vi "Scripting_AddVIInsideNoErrorCase.vi"(0 "ViToModify":refnum<vi>, 1 "VIToAdd":path=path "C:/GDS_Test/82/AO/NativeBase_class/protected/StartNP1.vi", 5 "error in (no error)":errorcluster, 6 "AddVIOnLeftSideCaseStructure":bool, 7 "OnlyReference":bool) -> (19 "error out":errorcluster)   [LabVIEW 2020]
uses:
  <vilib>/Utility/miscctls.llb/LVPointTypeDef.ctl
  <vilib>/Utility/miscctls.llb/LVPositionTypeDef.ctl
  <vilib>/Utility/miscctls.llb/LVRectTypeDef.ctl
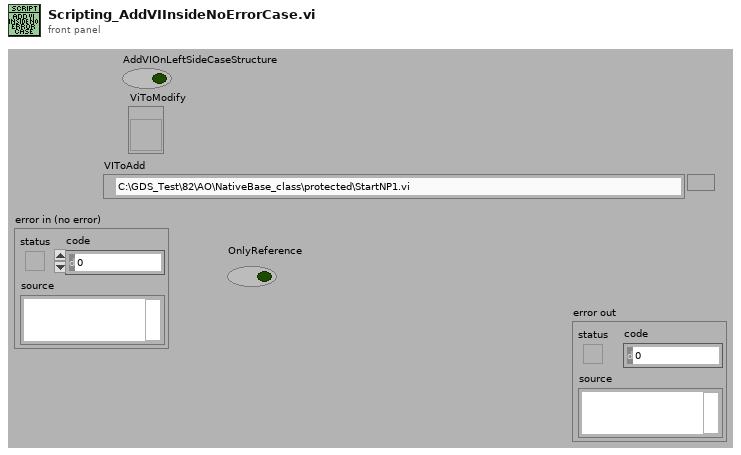
[diagram p1: front panel]
types:
  T1 = typedef "LVPositionTypeDef.ctl" = cluster{"Left":i32, "Top":i32}
  T2 = typedef "LVPointTypeDef.ctl" = cluster{"Horizontal":i16, "Vertical":i16}
  T3 = typedef "LVRectTypeDef.ctl" = cluster{"Left":i16, "Top":i16, "Right":i16, "Bottom":i16}
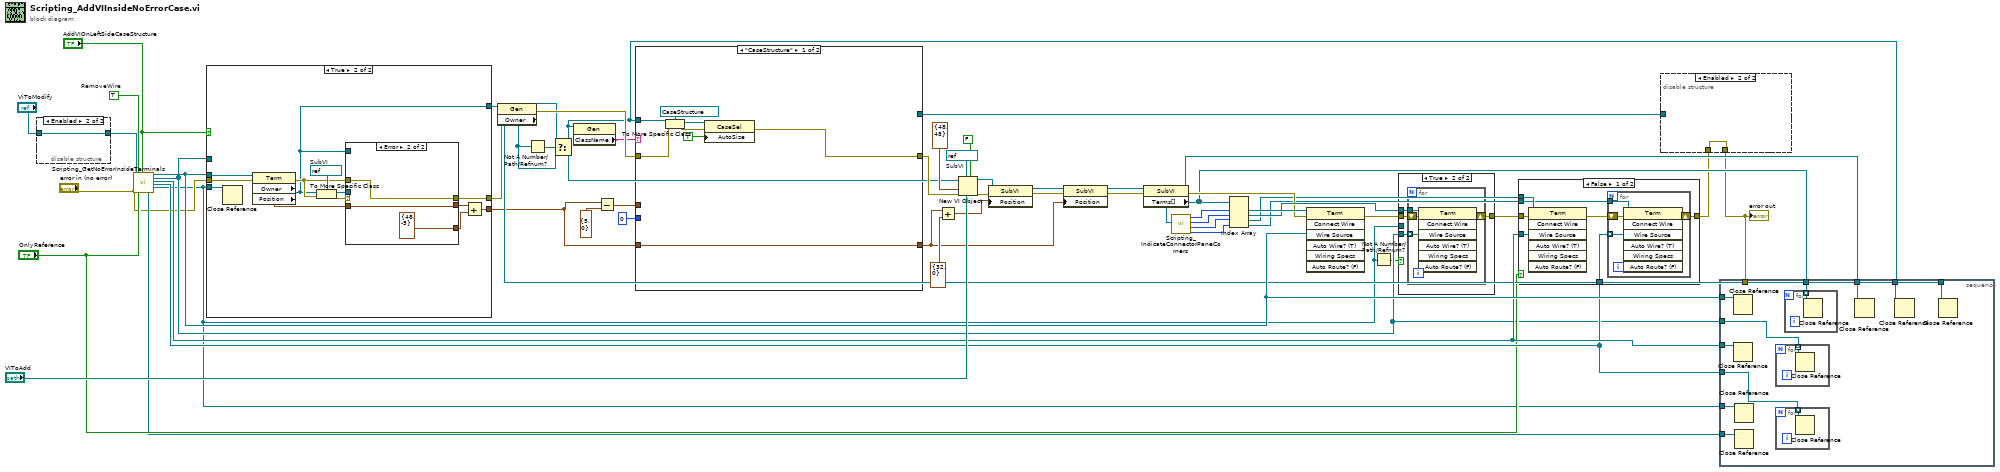
[diagram p0: block diagram]
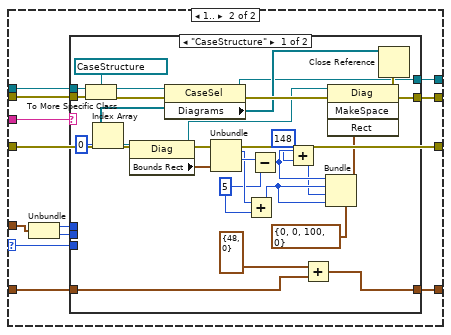
[diagram p3: hidden frame]
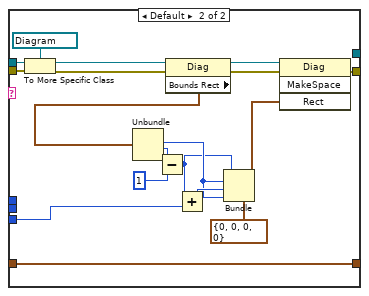
[diagram p4: hidden frame]
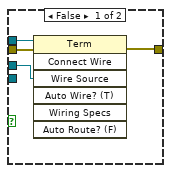
[diagram p5: hidden frame]
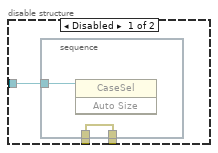
[diagram p6: hidden frame]
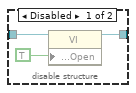
[diagram p7: hidden frame]
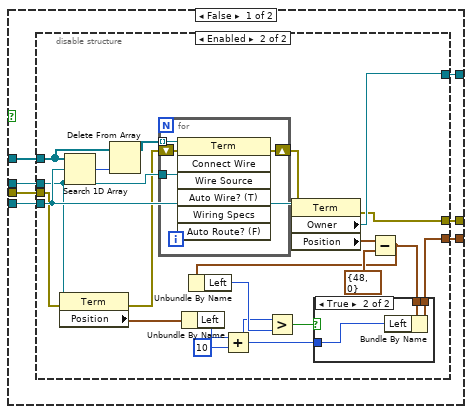
[diagram p9: hidden frame]
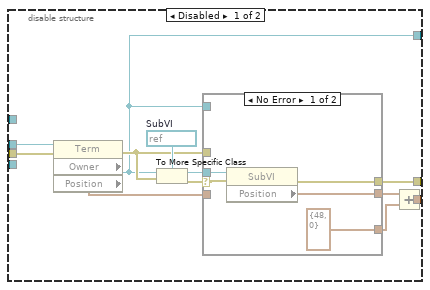
[diagram p10: hidden frame]
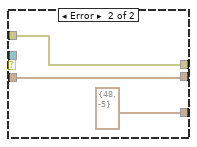
[diagram p11: hidden frame]
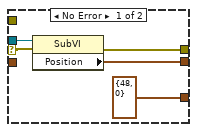
[diagram p13: hidden frame]
diagram:
  w51 = TRUE  # RemoveWire
  w55 = refnum<vi> refnum  # SubVI
  n1 = disable-structure shown="Enabled" {
    disable-tunnel: "ViToModify" -> [w58 w59]
    disable-tunnel: [w57 w59] -> w23
    frame Disabled {
      n2 = property class="VI"(reference=w58, "Front Panel.Open"=TRUE ("Front Panel Window:Open")) -> (reference out=w57:refnum<vi>)  [unwired: 1 in, 1 out]
    }
    frame Enabled {
    }
  }
  n3 = call <resource>:"Scripting_GetNoErrorInsideTerminals.vi"("ViReference"=w23, "error in (no error)"="error in (no error)", "RemoveWire(False)"=w51, "OnlyTop(False)"="OnlyReference", "GetCaseLeftTerminals(True)"="AddVIOnLeftSideCaseStructure") -> ("Bottom_InsideTermRefnumOut"=w12:refnum<vi>, "Top_WireTermSource"=w34:refnum<vi>, "Top_WireTermDrains"=w22:refnum<vi>[], "Bottom_WireTermSource"=w33:refnum<vi>, "Bottom_WireTermDrains"=w32:refnum<vi>[], "Top_InsideTermRefnumOut"=w9:refnum<vi>)  [unwired: 8 in, 1 out]
  n4 = case shown="True" "AddVIOnLeftSideCaseStructure" {
    tunnel: "error in (no error)" -> [w66 w127]
    tunnel: [w65 w120] -> w17
    tunnel: w34 -> [w64 w118]
    tunnel: [w63 w117] -> w37
    tunnel: [w62 w116] -> w29
    tunnel: w9 -> [w61 w115]
    tunnel: w22 -> [w60 _]
    frame False {
      n5 = disable-structure shown="Enabled" {
        disable-tunnel: w66 -> [w78 w96]
        disable-tunnel: [w72 w89] -> w65
        disable-tunnel: w64 -> [w70 w97]
        disable-tunnel: [w69 w103] -> w63
        disable-tunnel: [w68 w106] -> w62
        disable-tunnel: w61 -> [_ w102]
        disable-tunnel: w60 -> [_ w100]
        frame Disabled {
          w77 = refnum<vi> refnum  # SubVI
          n6 = property class="Term"(reference=w70, error in=w78) -> (error out=w71:errorcluster, "Owner"=w68:refnum<vi>, "Position"=w67:T1)  [unwired: 1 out]
          n7 = To More Specific Class(target class=w77, reference=w68, error in=w71) -> (specific class reference=w76:refnum<vi>, error out=w75:errorcluster)
          n8 = case shown="No Error" w75 {
            selector: w75 -> [w82 _]
            tunnel: w76 -> [w83 _]
            tunnel: w67 -> [_ w86]
            tunnel: [w81 w86] -> w74
            tunnel: [T1 {"Left"=48, "Top"=0} ("y") T1 {"Left"=48, "Top"=-5} ("y")] -> w73
            tunnel: [w79 w84] -> w69
            tunnel: w71 -> [_ w84]
            tunnel: w68 -> [_ _]
            frame No Error {
              n9 = property class="SubVI"(reference=w83, error in=w82) -> (error out=w79:errorcluster, "Position"=w81:T1)  [unwired: 1 out]
            }
            frame Error {
            }
          }
          n10 = Add(x=w74, y=w73) -> (x+y=w72:T1)
        }
        frame Enabled {
          n11 = property class="Term"(reference=w97, error in=w96) -> (error out=w95:errorcluster, "Position"=w94:T1)  [unwired: 1 out]
          n12 = Search 1D Array(1D array=w100, element=w102) -> (index of element=w101:i32)  [unwired: 1 in]
          n13 = Delete From Array(array=w100, index=w101) -> (array with subset deleted=w99:refnum<vi>[])  [unwired: 1 in, 1 out]
          n14 = for {
            tunnel: w99 -> [w114] mode=indexing
            tunnel: w97 -> [w113]
            shift-right: [w111] -> w98
            shift-left: w95 -> [w112]
            n15 = invoke class="Term" method="Connect Wire"(reference=w114, error in=w112, "Wire Source"=w113) -> (error out=w111:errorcluster)  [unwired: 4 in, 6 out]
          }
          n16 = Unbundle By Name(w94) -> ("Left"=w91:i32)
          n17 = Add(x=w91, y=10) -> (x+y=w87:i32)
          n18 = property class="Term"(reference=w102, error in=w98) -> (error out=w103:errorcluster, "Owner"=w106:refnum<vi>, "Position"=w105:T1)  [unwired: 1 out]
          n19 = Subtract(x=w105, y=T1 {"Left"=48, "Top"=0}) -> (x-y=w90:T1)
          n20 = Unbundle By Name(w90) -> ("Left"=w93:i32)
          n21 = Greater?(x=w87, y=w93) -> (0:w88:bool)
          n22 = case shown="True" w88 {
            tunnel: w90 -> [w107 w110]
            tunnel: [w107 w109] -> w89
            tunnel: w87 -> [_ w108]
            frame False {
            }
            frame True {
              n23 = Bundle By Name(cluster=w110, "Left"=w108) -> (w109:T1)
            }
          }
        }
      }
    }
    frame True {
      w126 = refnum<vi> refnum  # SubVI
      n24 = Close Reference(reference=w115) -> ()  [unwired: 1 in, 1 out]
      n25 = property class="Term"(reference=w118, error in=w127) -> (error out=w119:errorcluster, "Owner"=w116:refnum<vi>, "Position"=w123:T1)  [unwired: 1 out]
      n26 = To More Specific Class(target class=w126, reference=w116, error in=w119) -> (specific class reference=w125:refnum<vi>, error out=w124:errorcluster)
      n27 = case shown="Error" w124 {
        selector: w124 -> [w131 _]
        tunnel: w125 -> [w132 _]
        tunnel: w123 -> [_ w135]
        tunnel: [w130 w135] -> w122
        tunnel: [T1 {"Left"=48, "Top"=0} ("y") T1 {"Left"=48, "Top"=-5} ("y")] -> w121
        tunnel: [w128 w133] -> w117
        tunnel: w119 -> [_ w133]
        tunnel: w116 -> [_ _]
        frame No Error {
          n28 = property class="SubVI"(reference=w132, error in=w131) -> (error out=w128:errorcluster, "Position"=w130:T1)  [unwired: 1 out]
        }
        frame Error {
        }
      }
      n29 = Add(x=w122, y=w121) -> (x+y=w120:T1)
    }
  }
  n30 = property class="Gen"(reference=w29, error in=w37) -> (reference out=w27:refnum<vi>, error out=w35:errorcluster, "Owner"=w26:refnum<vi>)
  n31 = Not A Number/Path/Refnum?(number/path/refnum=w26) -> (NaN/Path/Refnum?=w28:bool)
  n32 = Select(t=w27, s=w28, f=w26) -> (s? t:f=w16:refnum<vi>)
  n33 = property class="Gen"(reference=w16) -> ("ClassName"=w8:string)  [unwired: 1 in, 2 out]
  n34 = Subtract(x=w17, y=T1 {"Left"=5, "Top"=0}) -> (x-y=w18:T1)
  n35 = case shown="\"CaseStructure\"" w8 {
    selector: w8 -> [_ w144]
    tunnel: [w137 w152] -> w36
    tunnel: w35 -> [w141 w151]
    tunnel: 0 -> [_ w150]
    tunnel: w18 -> [_ w149]
    tunnel: w17 -> [w136 w148]
    tunnel: [w136 w147] -> w1
    tunnel: w16 -> [w142 w146]
    tunnel: [_ w145] -> w15
    frame "CaseStructure" {
      n36 = To More Specific Class(target class=refnum<vi> refnum ("Block Diagram"), reference=w142, error in=w141) -> (specific class reference=w140:refnum<vi>, error out=w138:errorcluster)
      n37 = property class="CaseSel"(reference=w140, error in=w138, "AutoSize"=TRUE ("AutoSize To Fit Contents?")) -> (error out=w137:errorcluster)  [unwired: 1 out]
    }
    frame Default {
      n38 = case shown="Default" w150 {
        selector: w150 -> [_ w162]
        tunnel: w146 -> [_ w166]
        tunnel: [_ w165] -> _
        tunnel: w151 -> [w154 w164]
        tunnel: [w154 w164] -> w152
        tunnel: w151 -> [_ w163]
        tunnel: w149 -> [_ w161]
        tunnel: w144 -> [_ w160]
        tunnel: w148 -> [w153 w157]
        tunnel: [w153 w156] -> w147
        tunnel: [_ w155] -> w145
        frame Default {
        }
        frame 1.. {
          n39 = Unbundle(w161) -> ("Left"=w159:i32, "Top"=w158:i32)
          n40 = case shown="\"CaseStructure\"" w160 {
            tunnel: w166 -> [w190 w208]
            tunnel: [w179 w207] -> w165
            tunnel: w163 -> [w189 w206]
            tunnel: w162 -> [_ w199]
            tunnel: w159 -> [_ _]
            tunnel: w158 -> [_ _]
            tunnel: w157 -> [w169 w192]
            tunnel: [w168 w192] -> w156
            tunnel: [w167 _] -> w155
            frame "CaseStructure" {
              w175 = i16 5 ("y")
              n41 = To More Specific Class(target class=refnum<vi> refnum ("Block Diagram"), reference=w190, error in=w189) -> (specific class reference=w188:refnum<vi>, error out=w187:errorcluster)
              n42 = property class="CaseSel"(reference=w188, error in=w187) -> (reference out=w167:refnum<vi>, error out=w186:errorcluster, "Diagrams"=w178:refnum<vi>[])
              n43 = Index Array(array=w178, index=0) -> (element=w182:refnum<vi>)
              n44 = property class="Diag"(reference=w182) -> (reference out=w181:refnum<vi>, "Bounds Rect"=w180:T3)  [unwired: 1 in, 1 out]
              n45 = Unbundle(w180) -> ("Top"=w176:i16, "Right"=w183:i16)  [unwired: 2 out]
              n46 = Add(x=w176, y=w175) -> (x+y=w174:i16)
              n47 = Subtract(x=w183, y=w175) -> (x-y=w173:i16)
              n48 = Add(x=w173, y=i16 148 ("Right")) -> (x+y=w171:i16)
              n49 = Add(x=T1 {"Left"=48, "Top"=0} ("y"), y=w169) -> (x+y=w168:T1)
              n50 = Bundle(cluster=T3 {"Left"=0, "Top"=0, "Right"=100, "Bottom"=0} ("Rect"), "Left"=w173, "Top"=w174, "Right"=w171, "Bottom"=w174) -> (w184:T3)
              n51 = invoke class="Diag" method="MakeSpace"(reference=w181, error in=w186, "Rect"=w184) -> (error out=w179:errorcluster)  [unwired: 1 in, 3 out]
              n52 = Close Reference(reference=w178, error in (no error)=w179) -> ()  [unwired: 1 out]
            }
            frame Default {
              n53 = To More Specific Class(target class=refnum<vi> refnum ("Block Diagram"), reference=w208, error in=w206) -> (specific class reference=w205:refnum<vi>, error out=w204:errorcluster)
              n54 = property class="Diag"(reference=w205, error in=w204) -> (reference out=w203:refnum<vi>, error out=w202:errorcluster, "Bounds Rect"=w200:T3)
              n55 = Unbundle(w200) -> ("Top"=w196:i16, "Right"=w193:i16)  [unwired: 2 out]
              n56 = Subtract(x=w193, y=i16 1) -> (x-y=w194:i16)
              n57 = Add(x=w194, y=w199) -> (x+y=w198:i32)
              n58 = Bundle(cluster=T3 {"Left"=0, "Top"=0, "Right"=0, "Bottom"=0} ("Rect"), "Left"=w194, "Top"=w196, "Right"=w198, "Bottom"=w196) -> (w197:T3)
              n59 = invoke class="Diag" method="MakeSpace"(reference=w203, error in=w202, "Rect"=w197) -> (error out=w207:errorcluster)  [unwired: 1 in, 3 out]
            }
          }
        }
      }
    }
  }
  n60 = Add(x=w1, y=T1 {"Left"=32, "Top"=0}) -> (x+y=w2:T1)
  n61 = New VI Object(vi object class=w55, auto wire? (F)=FALSE, owner refnum=w16, position/next to=T2 {"Horizontal"=48, "Vertical"=48} ("relative position/next to refnum"), 6:"VIToAdd", 8:w36) -> (object refnum=w52:refnum<vi>, 0:w53:errorcluster)  [unwired: 2 in]
  n62 = property class="SubVI"(reference=w52, error in=w53, "Position"=w2) -> (reference out=w7:refnum<vi>, error out=w6:errorcluster)
  n63 = property class="SubVI"(reference=w7, error in=w6, "Position"=w1) -> (reference out=w5:refnum<vi>, error out=w4:errorcluster)
  n64 = property class="SubVI"(reference=w5, error in=w4) -> (reference out=w30:refnum<vi>, error out=w44:errorcluster, "Terms[]"=w31:refnum<vi>[])
  n65 = call <resource>:"Scripting_IndicateConnectorPaneCorners.vi"("Terminals[]"=w31) -> ("RightLower"=w41:i32, "LeftLower"=w42:i32, "RightTop"=w48:i32, "LeftTop"=w49:i32)  [unwired: 7 in]
  n66 = Index Array(array=w31, index #1=w49, index #2=w48, index #3=w42, index #4=w41) -> (element #1=w47:refnum<vi>, element #2=w46:refnum<vi>, element #3=w40:refnum<vi>, element #4=w39:refnum<vi>)
  n67 = invoke class="Term" method="Connect Wire"(reference=w47, error in=w44, "Wire Source"=w34) -> (error out=w45:errorcluster)  [unwired: 4 in, 6 out]
  n68 = Not A Number/Path/Refnum?(number/path/refnum=w9) -> (NaN/Path/Refnum?=w10:bool)
  n69 = case shown="True" w10 {
    tunnel: w46 -> [w211 w217]
    tunnel: w45 -> [w213 w216]
    tunnel: [w210 w215] -> w43
    tunnel: w22 -> [_ w214]
    tunnel: w9 -> [w212 _]
    frame False {
      n70 = invoke class="Term" method="Connect Wire"(reference=w211, error in=w213, "Wire Source"=w212) -> (error out=w210:errorcluster)  [unwired: 4 in, 6 out]
    }
    frame True {
      n71 = for {
        tunnel: w217 -> [w221]
        tunnel: w214 -> [w218] mode=indexing
        shift-right: [w219] -> w215
        shift-left: w216 -> [w220]
        n72 = invoke class="Term" method="Connect Wire"(reference=w221, error in=w220, "Wire Source"=w218) -> (error out=w219:errorcluster)  [unwired: 4 in, 6 out]
      }
    }
  }
  n73 = case shown="False" "OnlyReference" {
    tunnel: w43 -> [w228 w233]
    tunnel: w40 -> [w227 _]
    tunnel: w39 -> [w226 _]
    tunnel: [w224 w233] -> w14
    tunnel: w33 -> [w223 _]
    tunnel: w32 -> [w222 _]
    frame False {
      n74 = invoke class="Term" method="Connect Wire"(reference=w227, error in=w228, "Wire Source"=w223) -> (error out=w225:errorcluster)  [unwired: 4 in, 6 out]
      n75 = for {
        tunnel: w226 -> [w232]
        tunnel: w222 -> [w229] mode=indexing
        shift-right: [w230] -> w224
        shift-left: w225 -> [w231]
        n76 = invoke class="Term" method="Connect Wire"(reference=w232, error in=w231, "Wire Source"=w229) -> (error out=w230:errorcluster)  [unwired: 4 in, 6 out]
      }
    }
    frame True {
    }
  }
  n77 = disable-structure shown="Enabled" {
    disable-tunnel: w15 -> [w236 _]
    disable-tunnel: w14 -> [w235 w239]
    disable-tunnel: [w234 w239] -> w13
    frame Disabled {
      n78 = stacked-sequence {
        tunnel: w235 -> [w237]
        tunnel: w236 -> [w238]
        tunnel: [w237] -> w234
        frame #0 {
          n79 = invoke class="CaseSel" method="Auto Size"(reference=w238) -> ()  [unwired: 2 in, 3 out]
        }
      }
    }
    frame Enabled {
    }
  }
  "error out" <- w13
  n80 = stacked-sequence {
    tunnel: w13 -> [_]
    tunnel: w34 -> [w249]
    tunnel: w22 -> [w243]
    tunnel: w33 -> [w248]
    tunnel: w32 -> [w242]
    tunnel: w31 -> [w247]
    tunnel: w30 -> [w246]
    tunnel: w29 -> [w245]
    tunnel: w16 -> [w244]
    tunnel: w12 -> [w241]
    tunnel: w9 -> [w240]
    frame #0 {
      n81 = Close Reference(reference=w249) -> ()  [unwired: 1 in, 1 out]
      n82 = Close Reference(reference=w248) -> ()  [unwired: 1 in, 1 out]
      n83 = Close Reference(reference=w240) -> ()  [unwired: 1 in, 1 out]
      n84 = Close Reference(reference=w241) -> ()  [unwired: 1 in, 1 out]
      n85 = for {
        tunnel: w243 -> [w251] mode=indexing
        n86 = Close Reference(reference=w251) -> ()  [unwired: 1 in, 1 out]
      }
      n87 = for {
        tunnel: w242 -> [w250] mode=indexing
        n88 = Close Reference(reference=w250) -> ()  [unwired: 1 in, 1 out]
      }
      n89 = for {
        tunnel: w247 -> [w252] mode=indexing
        n90 = Close Reference(reference=w252) -> ()  [unwired: 1 in, 1 out]
      }
      n91 = Close Reference(reference=w246) -> ()  [unwired: 1 in, 1 out]
      n92 = Close Reference(reference=w244) -> ()  [unwired: 1 in, 1 out]
      n93 = Close Reference(reference=w245) -> ()  [unwired: 1 in, 1 out]
    }
  }
